vi "Batch Enable Controls.vi"(7 "Enabled State":T1(ring), 8 "error in (no error)":errorcluster, 11 "GObject:Control Refnums":refnum<vi>[](array[refnum])) -> (0 "error out":errorcluster)   [LabVIEW 8.6]
doc: "This function enables, disables, and disables-and-greys-out a set of controls and indicators en masse. Its input is an array of \"GOjbect:Control\" refnums."
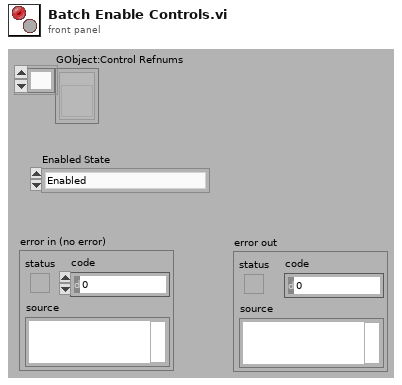
[diagram p1: front panel]
types:
  T1 = enum8{"Enabled", "Disabled", "Disabled and Grayed Out"}
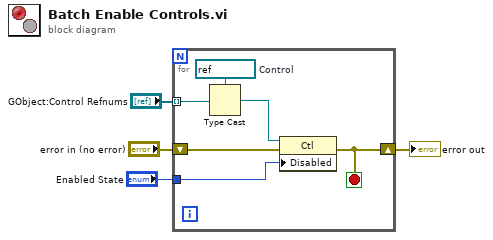
[diagram p0: block diagram]
diagram:
  n1 = for {
    tunnel: "GObject:Control Refnums" -> [w7] mode=indexing
    shift-right: [w9] -> w2
    shift-left: "error in (no error)" -> [w10]
    tunnel: "Enabled State" -> [w5]
    stop <- w9 stop-if-true
    w8 = refnum<vi> ?  # Control
    n2 = Type Cast(type=w8, x=w7) -> (*(type *) &x=w6:refnum<vi>)
    n3 = property on="Property Node" class="Ctl"(reference=w6, error in=w10, "Disabled"=w5) -> (error out=w9:errorcluster)  [unwired: 1 out]
  }
  "error out" <- w2
